vi "Keithley24xx_qMeasVih.vi"(3 "Vol, V":dbl, 4 "Vih, V":dbl, 5 "Vil, V":dbl, 6 "outErr In":errorcluster, 8 "outVISA In":refnum<visa-resource-name>, 9 "inVISA In":refnum<visa-resource-name>, 11 "inErr In":errorcluster) -> (0 "outVISA Out":refnum<visa-resource-name>, 1 "inErr Out":errorcluster, 2 "Vih meas, В":dbl format="%#.3g", 7 "inVISA Out":refnum<visa-resource-name>, 10 "outErr Out":errorcluster)   [LabVIEW 2014]
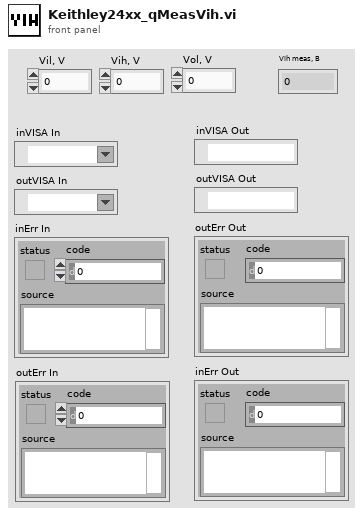
[diagram p1: front panel]
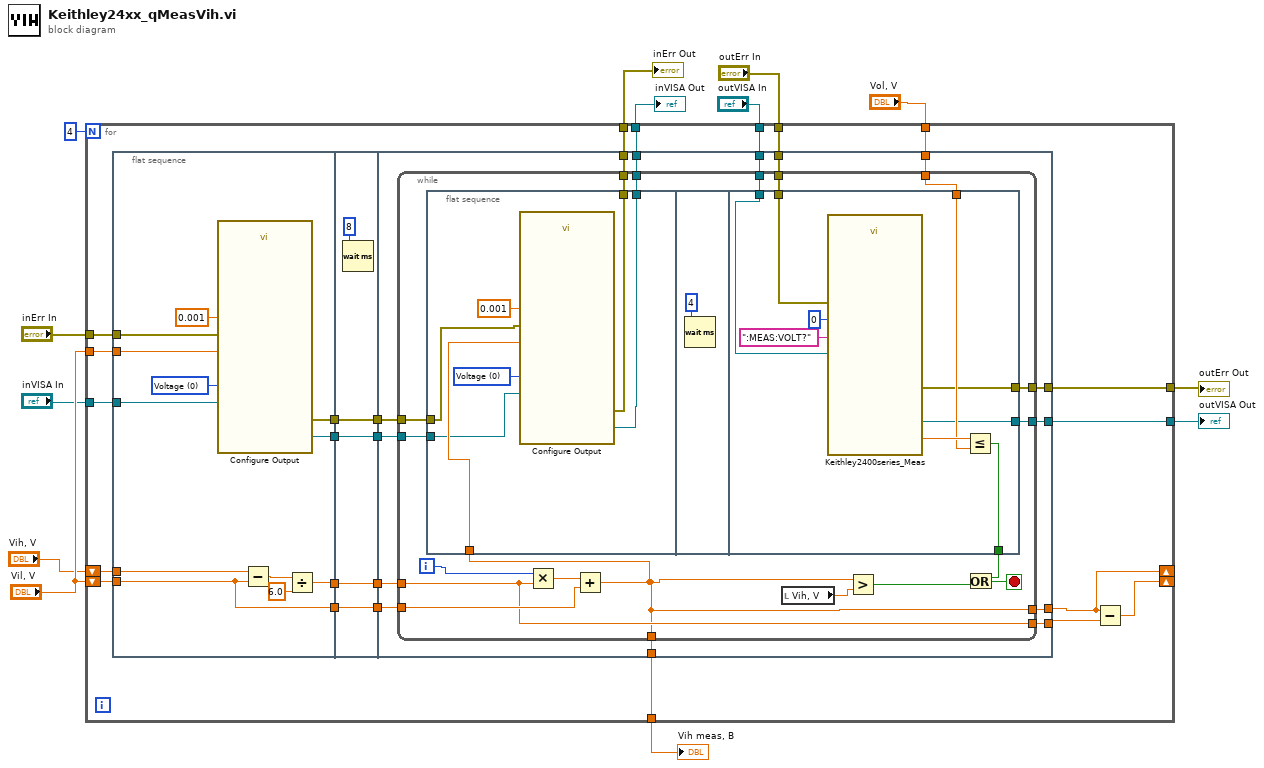
[diagram p0: block diagram]
diagram:
  n1 = for {
    N: 4 -> [_]
    shift-right: [w29] -> _
    shift-left: "Vil, V" -> [w35]
    shift-right: [w28] -> _
    shift-left: "Vih, V" -> [w34]
    tunnel: "Vil, V" -> [w33]
    tunnel: "Vol, V" -> [w27]
    tunnel: "inVISA In" -> [w26]
    tunnel: "inErr In" -> [w25]
    tunnel: [w20] -> w7
    tunnel: [w19] -> w6
    tunnel: "outVISA In" -> [w18]
    tunnel: "outErr In" -> [w17]
    tunnel: [w16] -> w2
    tunnel: [w15] -> w3
    tunnel: [w14] -> w1
    n2 = flat-sequence {
      tunnel: [w45] -> w37
      tunnel: w35 -> [w42]
      tunnel: w34 -> [w44]
      tunnel: w33 -> [w43]
      tunnel: [w42] -> w32
      tunnel: w26 -> [w41]
      tunnel: w25 -> [w40]
      tunnel: [w39] -> w23
      tunnel: [w38] -> w21
      tunnel: w37 -> [w53]
      tunnel: [w53] -> w36
      tunnel: w32 -> [w52]
      tunnel: [w52] -> w31
      tunnel: [w51] -> w24
      tunnel: w23 -> [w51]
      tunnel: [w50] -> w22
      tunnel: w21 -> [w50]
      tunnel: w36 -> [w68]
      tunnel: w31 -> [w67]
      tunnel: [w66] -> w28
      tunnel: [w65] -> w30
      tunnel: w27 -> [w64]
      tunnel: w24 -> [w63]
      tunnel: w22 -> [w62]
      tunnel: [w61] -> w20
      tunnel: [w60] -> w19
      tunnel: w18 -> [w59]
      tunnel: w17 -> [w58]
      tunnel: [w57] -> w16
      tunnel: [w56] -> w15
      tunnel: [w55] -> w14
      frame #0 {
        w49 = u16 0 items=["Voltage", "Current"] ("Source Mode  (0: Voltage)")
        n3 = call "Configure Output.vi"("Source Mode  (0: Voltage)"=w49, "error in (no error)"=w40, "Compliance  Level (0.1)"=0.001, "Output Level (0)"=w43, "VISA resource name"=w41) -> ("error out"=w38:errorcluster, "VISA resource name out"=w39:refnum<visa-resource-name>)  [unwired: 5 in]
        n4 = Subtract(x=w44, y=w42) -> (x-y=w47:dbl)
        n5 = Divide(x=w47, y=6.0) -> (x/y=w45:dbl)
      }
      frame #1 {
        n6 = Wait (ms)(milliseconds to wait=u32 8) -> ()  [unwired: 1 out]
      }
      frame #2 {
        n7 = while {
          tunnel: w68 -> [w79]
          tunnel: w67 -> [w81]
          tunnel: [w69] -> w66
          tunnel: [w79] -> w65
          tunnel: w64 -> [w78]
          tunnel: w63 -> [w77]
          tunnel: w62 -> [w76]
          tunnel: [w75] -> w61
          tunnel: [w74] -> w60
          tunnel: w59 -> [w73]
          tunnel: w58 -> [w72]
          tunnel: [w71] -> w57
          tunnel: [w70] -> w56
          tunnel: [w69] -> w55
          i -> [w82]
          stop <- w85 stop-if-true
          n8 = flat-sequence {
            tunnel: w69 -> [w92]
            tunnel: w77 -> [w91]
            tunnel: w76 -> [w90]
            tunnel: [w89] -> w75
            tunnel: [w88] -> w74
            tunnel: [w100] -> w84
            tunnel: w78 -> [w99]
            tunnel: w73 -> [w98]
            tunnel: w72 -> [w97]
            tunnel: [w96] -> w71
            tunnel: [w95] -> w70
            frame #0 {
              w93 = u16 0 items=["Voltage", "Current"] ("Source Mode  (0: Voltage)")
              n9 = call "Configure Output.vi"("Source Mode  (0: Voltage)"=w93, "error in (no error)"=w90, "Compliance  Level (0.1)"=0.001, "Output Level (0)"=w92, "VISA resource name"=w91) -> ("error out"=w89:errorcluster, "VISA resource name out"=w88:refnum<visa-resource-name>)  [unwired: 5 in]
            }
            frame #1 {
              n10 = Wait (ms)(milliseconds to wait=u32 4) -> ()  [unwired: 1 out]
            }
            frame #2 {
              n11 = call "Keithley2400series_Meas.vi"("MEAS:<f>"=":MEAS:VOLT?", "error in (no error)"=w97, "MEAS mode, 0 Volt"=u16 0, "VISA resource name in"=w98) -> ("error out"=w95:errorcluster, "Замер"=w101:dbl, "VISA out"=w96:refnum<visa-resource-name>)  [unwired: 1 in, 1 out]
              n12 = Less Or Equal?(x=w101, y=w99) -> (x <= y?=w100:bool)
            }
          }
          n13 = Multiply(x=w82, y=w79) -> (x*y=w86:dbl)
          n14 = Add(x=w86, y=w81) -> (x+y=w69:dbl)
          n15 = local read "Vih, V"() -> (w80:dbl)
          n16 = Greater?(x=w69, y=w80) -> (0:w83:bool)
          n17 = Or(x=w84, y=w83) -> (x .or. y?=w85:bool)
        }
      }
    }
    n18 = Subtract(x=w28, y=w30) -> (x-y=w29:dbl)
  }
  "Vih meas, В" <- w1
  "inVISA Out" <- w6
  "outVISA Out" <- w2
  "outErr Out" <- w3
  "inErr Out" <- w7
